vi "Add Device.vi"(8 "error in (no error)":errorcluster, 10 "Device Model":refnum<class "Device.lvclass">, 11 "HAL Manager in":refnum<class "HAL Manager.lvclass">) -> (0 "error out":errorcluster, 2 "Device":refnum<class "Device.lvclass">, 3 "HAL Manager out":refnum<class "HAL Manager.lvclass">)   [LabVIEW 2012, in "HAL.lvlib" / "HAL Manager.lvclass"]
doc: "When programmatically creating device instances, they need to be added to a manager instance before calling the other device VIs on the manager. Since the base Device class needs to be in the 'Initialized' state to track its name in the future if not already set, this VI will call the Ctor VI on the device to initialize the instance. Devices in any state can be added to the manager instance."
uses:
  HAL Manager.lvclass
  Device/Device.lvclass
  <vilib>/ErrorRing/Error Ring.xnode
  <vilib>/Utility/error.llb/Error Cluster From Error Code.vi
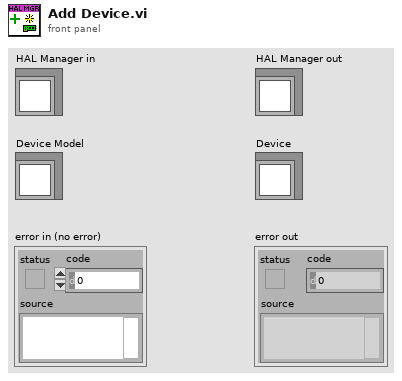
[diagram p1: front panel]
types:
  T1 = typedef "HAL.lvlib/Device.lvclass/Device State.ctl" = enum16{"Uninitialized", "Initialized", "Ready", "Running", "Error"}
  T2 = typedef "HAL.lvlib/HAL Manager.lvclass/Ref Data.ctl" = cluster{"Devices":refnum<class "Device.lvclass">[], "Type":string[], "Models":string[], "Name":string[]}
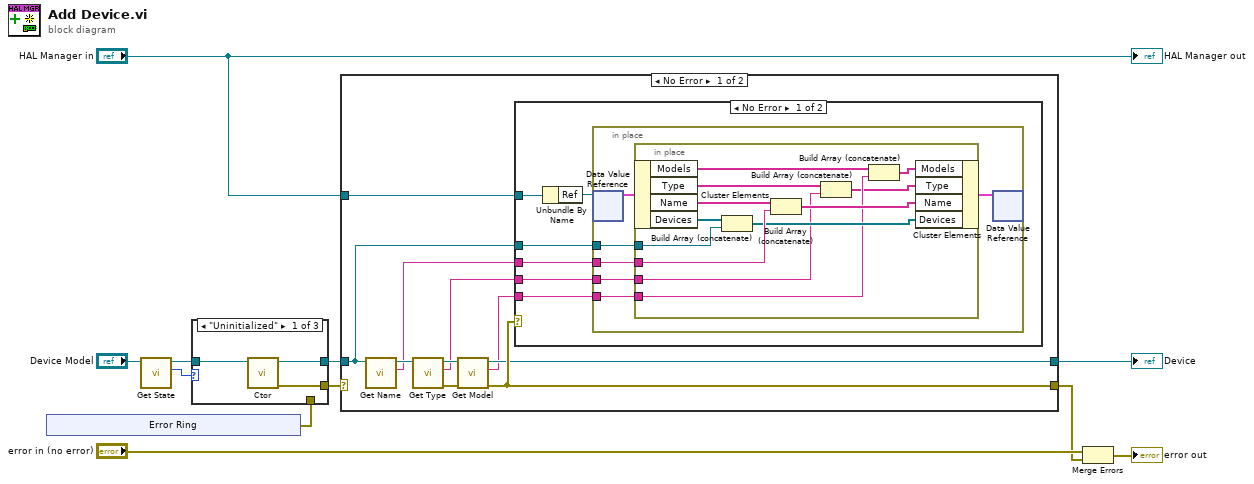
[diagram p0: block diagram]
diagram:
  n1 = xnode "Error Ring"() -> ("error out"=w7:errorcluster)
  n2 = call "Get State.vi"("Device in"="Device Model") -> ("Device State"=w8:T1, "Device out"=w9:refnum<class "Device.lvclass">)  [unwired: 8 in, 1 out]
  n3 = case shown="\"Uninitialized\"" w8 {
    tunnel: w9 -> [w14 w15 w17]
    tunnel: [w13 w15 w17] -> w5
    tunnel: w7 -> [_ _ w16]
    tunnel: [w12 _ w16] -> w6
    frame "Uninitialized" {
      n4 = call "Ctor.vi"("Device in"=w14) -> ("error out"=w12:errorcluster, "Device out"=w13:refnum<class "Device.lvclass">)  [unwired: 9 in]
    }
    frame Default {
    }
    frame "Error" {
    }
  }
  n5 = case shown="No Error" w6 {
    selector: w6 -> [_ w52]
    tunnel: w5 -> [w22 w53]
    tunnel: "HAL Manager in" -> [w20 _]
    tunnel: [w19 w53] -> w4
    tunnel: [w24 w52] -> w2
    frame No Error {
      n6 = call "Get Name.vi"("Device in"=w22) -> ("Name"=w21:string, "Device out"=w27:refnum<class "Device.lvclass">)  [unwired: 8 in, 1 out]
      n7 = call-dynamic "Get Type.vi"("Device in"=w27) -> ("error out"=w26:errorcluster, "Type"=w23:string, "Device out"=w25:refnum<class "Device.lvclass">)  [unwired: 8 in]
      n8 = call-dynamic "Get Model.vi"("error in (no error)"=w26, "Device in"=w25) -> ("error out"=w24:errorcluster, "Model"=w18:string, "Device out"=w19:refnum<class "Device.lvclass">)  [unwired: 7 in]
      n9 = case shown="No Error" w24 {
        tunnel: w18 -> [w28 _]
        tunnel: w22 -> [w31 _]
        tunnel: w23 -> [w29 _]
        tunnel: w21 -> [w30 _]
        tunnel: w20 -> [w32 _]
        frame No Error {
          n10 = Unbundle By Name(w32) -> ("Ref"=w33:refnum<data-value>)
          n11 = in-place {
            in-place-border: w31 -> [w37]
            in-place-border: w30 -> [w36]
            in-place-border: w29 -> [w35]
            in-place-border: w28 -> [w34]
            n12 = in-place-dvr #1(w33) -> (w39:T2)  [unwired: 1 out]
            n13 = in-place {
              in-place-border: w37 -> [w50]
              in-place-border: w36 -> [w48]
              in-place-border: w35 -> [w44]
              in-place-border: w34 -> [w42]
              n14 = in-place-cluster #2(w39) -> ("Models"=w43:string[], "Type"=w45:string[], "Name"=w49:string[], "Devices"=w51:refnum<class "Device.lvclass">[])
              n15 = Build Array (concatenate)(w51, w50) -> (w47:refnum<class "Device.lvclass">[])
              n16 = Build Array (concatenate)(w49, w48) -> (w46:string[])
              n17 = Build Array (concatenate)(w45, w44) -> (w40:string[])
              n18 = Build Array (concatenate)(w43, w42) -> (w41:string[])
              n19 = in-place-cluster #2("Models"=w41, "Type"=w40, "Name"=w46, "Devices"=w47) -> (w38:T2)
            }
            n20 = in-place-dvr #1(w38) -> ()  [unwired: 2 out]
          }
        }
        frame Error {
        }
      }
    }
    frame Error {
    }
  }
  "Device" <- w4
  n21 = Merge Errors("error in (no error)", w2) -> (→"error out":errorcluster)
  "HAL Manager out" <- "HAL Manager in"
